vi "CRYTree Manipulate Sub.vi"(6 "Type":enum16{"Curves", "Values", "Results", "WFM"}(ring), 7 "sAction":string, 8 "sData":string[](array[string]), 9 "nData":i32[](array[numeric]), 10 "sOption":string, 11 "Tree in":refnum<vi>) -> (0 "bData out":bool, 1 "sData Out":string[](array[string]), 2 "bOnlyGroup":bool, 3 "Tree Out":refnum<vi>, 4 "bCategory":bool)   [LabVIEW 2013]
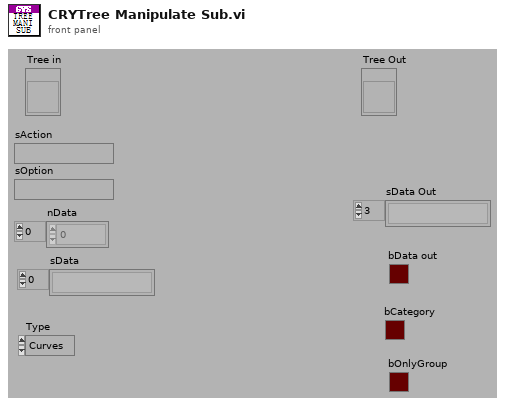
[diagram p1: front panel]
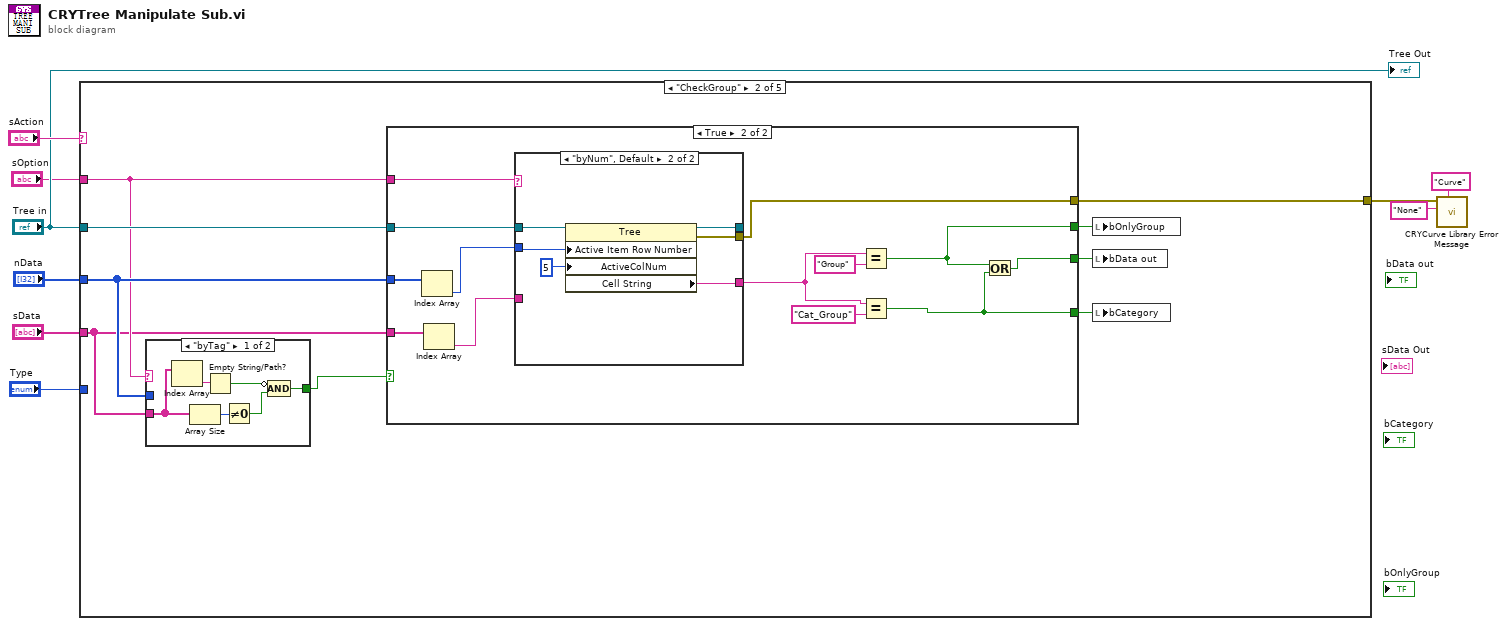
[diagram p0: block diagram]
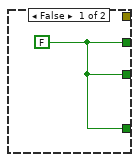
[diagram p3: hidden frame]
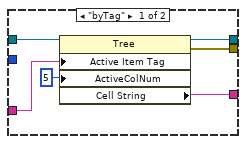
[diagram p4: hidden frame]
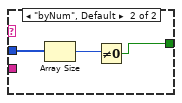
[diagram p5: hidden frame]
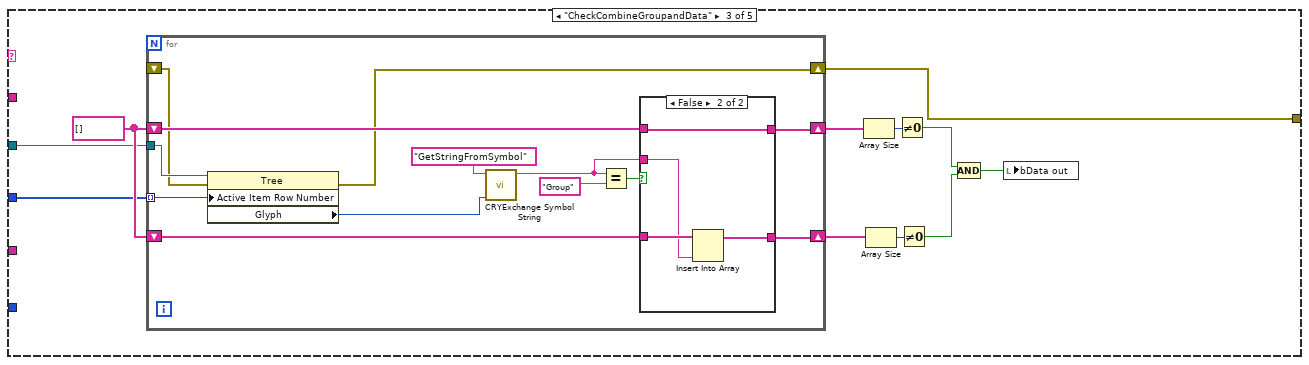
[diagram p6: hidden frame]
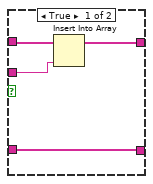
[diagram p7: hidden frame]
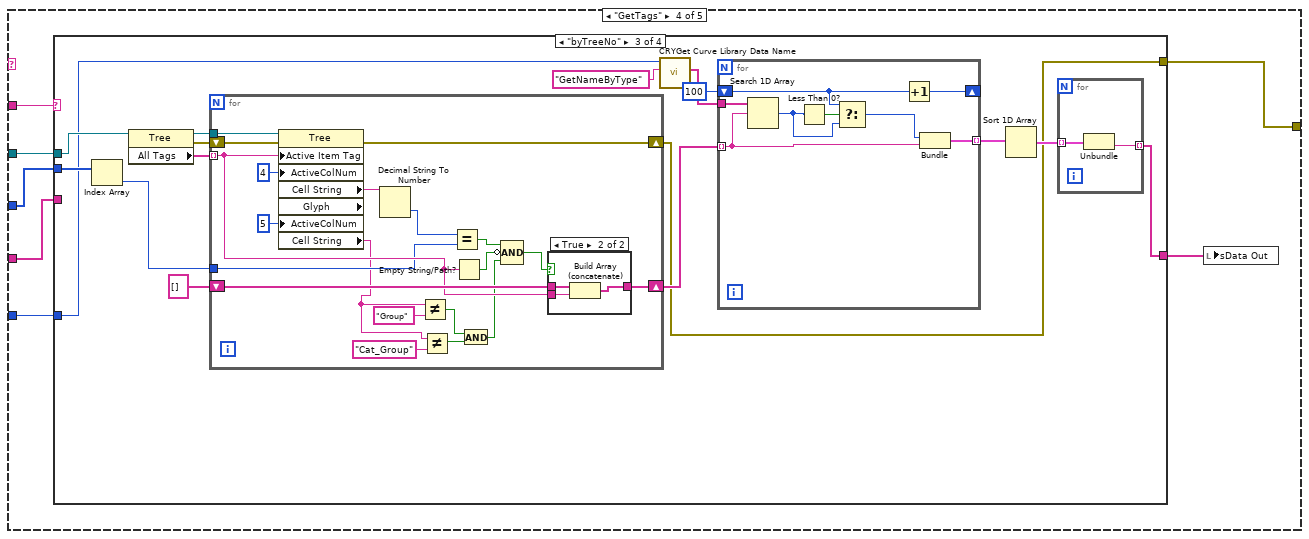
[diagram p8: hidden frame]
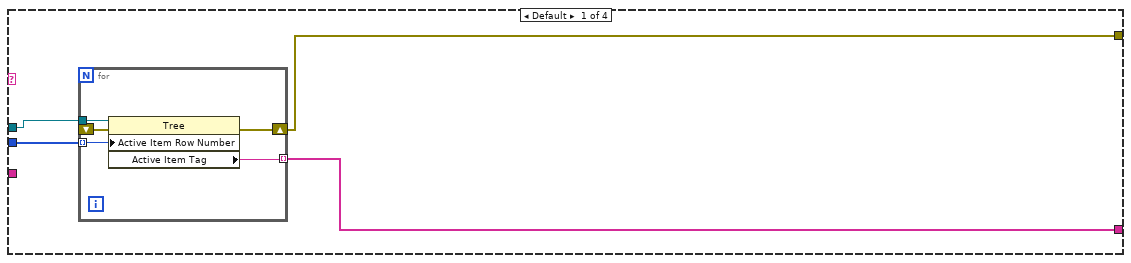
[diagram p9: hidden frame]
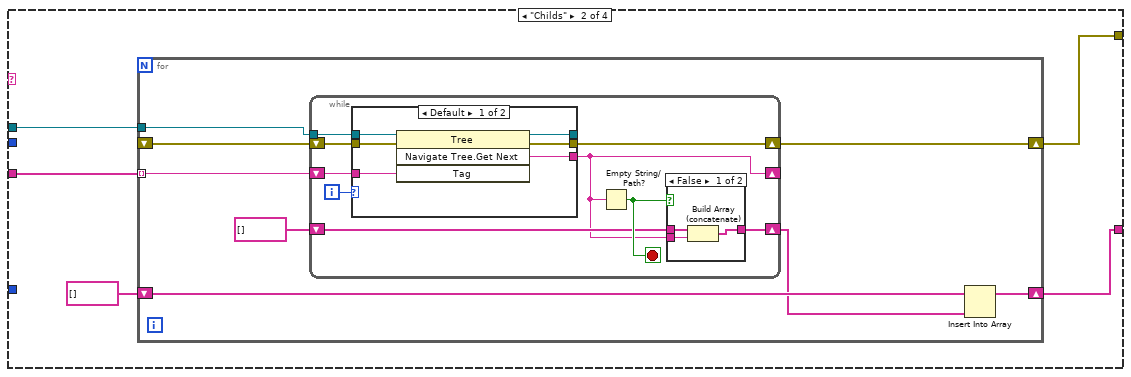
[diagram p10: hidden frame]
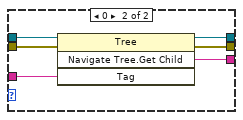
[diagram p12: hidden frame]
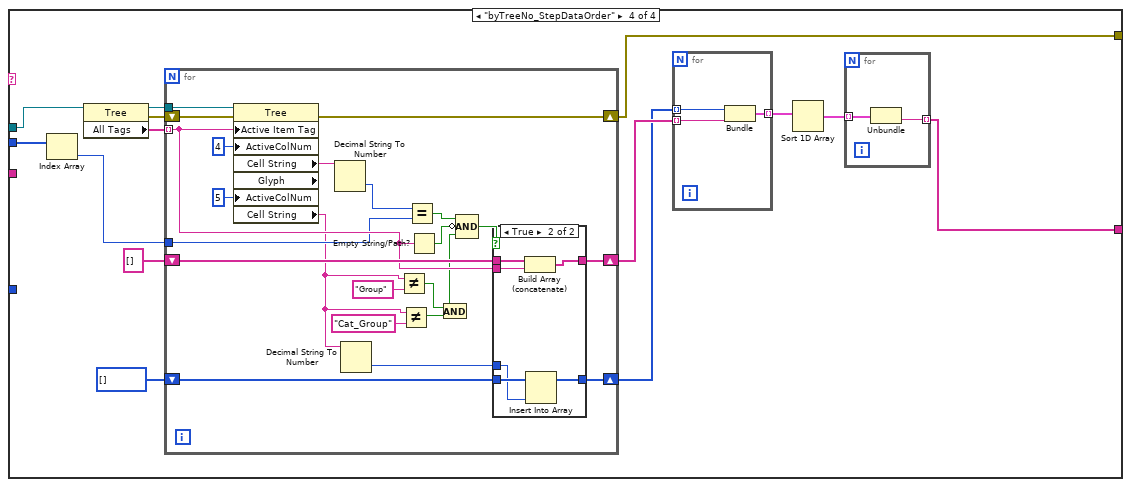
[diagram p14: hidden frame]
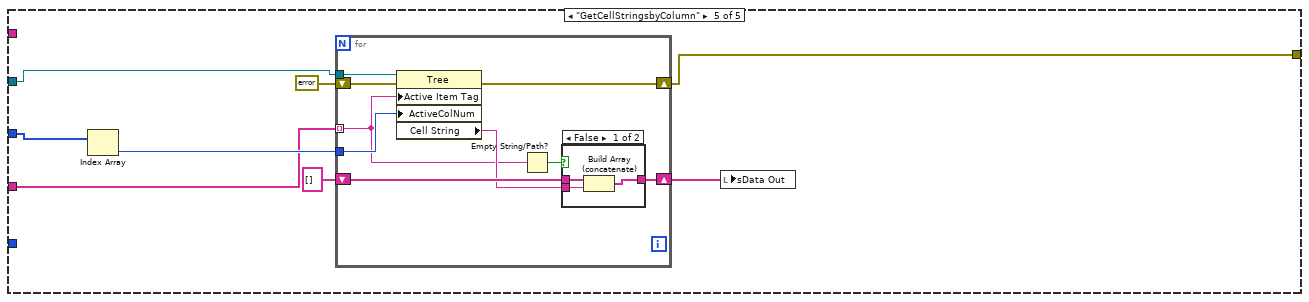
[diagram p16: hidden frame]
diagram:
  n1 = case shown="\"CheckGroup\"" "sAction" {
    tunnel: "nData" -> [_ w14 w55 w91 w245]
    tunnel: "Tree in" -> [_ w18 w56 w90 w242]
    tunnel: "sData" -> [_ w12 _ w89 w243]
    tunnel: "sOption" -> [_ w13 _ w88 _]
    tunnel: "Type" -> [_ _ _ w87 _]
    tunnel: [_ w10 w54 w86 w240] -> w1
    frame Default {
    }
    frame "CheckGroup" {
      n2 = case shown="\"byTag\"" w13 {
        tunnel: w12 -> [w48 _]
        tunnel: [w45 w51] -> w11
        tunnel: w14 -> [_ w53]
        frame "byTag" {
          n3 = Index Array(array=w48) -> (element=w49:string)  [unwired: 1 in]
          n4 = Array Size(array=w48) -> (size(s)=w47:i32)
          n5 = Empty String/Path?(string/path=w49) -> (empty?=w50:bool)
          n6 = Not Equal To 0?(x=w47) -> (x != 0?=w46:bool)
          n7 = Compound Arithmetic op=AND(invert w50, w46) -> (w45:bool)
        }
        frame "byNum", Default {
          n8 = Array Size(array=w53) -> (size(s)=w52:i32)
          n9 = Not Equal To 0?(x=w52) -> (x != 0?=w51:bool)
        }
      }
      n10 = case shown="True" w11 {
        tunnel: w18 -> [_ w31]
        tunnel: w13 -> [_ w30]
        tunnel: [w19 w29] -> w17
        tunnel: [w19 w27] -> w16
        tunnel: [w19 w26] -> w15
        tunnel: w12 -> [_ w22]
        tunnel: w14 -> [_ w21]
        tunnel: [_ w20] -> w10
        frame False {
          w19 = FALSE
        }
        frame True {
          n11 = Index Array(array=w21) -> (element=w25:i32)  [unwired: 1 in]
          n12 = Index Array(array=w22) -> (element=w24:string)  [unwired: 1 in]
          n13 = case shown="\"byNum\", Default" w30 {
            tunnel: w31 -> [w38 w44]
            tunnel: [w37 w43] -> _
            tunnel: w25 -> [_ w40]
            tunnel: [w35 w41] -> w23
            tunnel: w24 -> [w34 _]
            tunnel: [w33 w39] -> w20
            frame "byTag" {
              n14 = property class="Tree"(reference=w38, "Active Item Tag"=w34, "ActiveColNum"=5 ("Active Cell:Active Column Number")) -> (reference out=w37:refnum<vi>, error out=w33:errorcluster, "Cell String"=w35:string)  [unwired: 1 in]
            }
            frame "byNum", Default {
              n15 = property class="Tree"(reference=w44, "Active Item Row Number"=w40, "ActiveColNum"=5 ("Active Cell:Active Column Number")) -> (reference out=w43:refnum<vi>, error out=w39:errorcluster, "Cell String"=w41:string)  [unwired: 1 in]
            }
          }
          n16 = Equal?(x=w23, y="Group" ("sData out")) -> (x = y?=w29:bool)
          n17 = Equal?(x=w23, y="Cat_Group" ("sData out")) -> (x = y?=w26:bool)
          n18 = Or(x=w29, y=w26) -> (x .or. y?=w27:bool)
        }
      }
      n19 = local write "bOnlyGroup"(w17) -> ()
      n20 = local write "bData out"(w16) -> ()
      n21 = local write "bCategory"(w15) -> ()
    }
    frame "CheckCombineGroupandData" {
      w64 = string[] []
      n22 = for {
        tunnel: w55 -> [w71] mode=indexing
        shift-right: [w74] -> w63
        shift-left: w64 -> [w75]
        shift-right: [w72] -> w60
        shift-left: w64 -> [w73]
        tunnel: w56 -> [w69]
        shift-right: [w66] -> w54
        shift-left: _ -> [w65]
        n23 = property class="Tree"(reference=w69, error in=w65, "Active Item Row Number"=w71) -> (error out=w66:errorcluster, "Glyph"=w70:i32)  [unwired: 1 out]
        n24 = call "CRYExchange Symbol String.vi"("nData"=w70, "sAction"="GetStringFromSymbol") -> ("sData out"=w68:string)  [unwired: 8 in, 1 out]
        n25 = Equal?(x=w68, y="Group" ("sData out")) -> (x = y?=w67:bool)
        n26 = case shown="False" w67 {
          tunnel: w68 -> [w79 w83]
          tunnel: w75 -> [w81 w82]
          tunnel: [w80 w82] -> w74
          tunnel: w73 -> [w78 w85]
          tunnel: [w78 w84] -> w72
          frame True {
            n27 = Insert Into Array(array=w81, new element=w79) -> (w80:string[])  [unwired: 1 in]
          }
          frame False {
            n28 = Insert Into Array(array=w85, new element=w83) -> (w84:string[])  [unwired: 1 in]
          }
        }
      }
      n29 = Array Size(array=w63) -> (size(s)=w62:i32)
      n30 = Array Size(array=w60) -> (size(s)=w61:i32)
      n31 = Not Equal To 0?(x=w62) -> (x != 0?=w59:bool)
      n32 = Not Equal To 0?(x=w61) -> (x != 0?=w58:bool)
      n33 = Compound Arithmetic op=AND(w59, w58) -> (w57:bool)
      n34 = local write "bData out"(w57) -> ()
    }
    frame "GetTags" {
      n35 = case shown="\"byTreeNo\"" w88 {
        tunnel: [w95 w106 w144 w194] -> w92
        tunnel: w91 -> [w94 _ w155 w203]
        tunnel: w90 -> [w96 w105 w152 w200]
        tunnel: w89 -> [_ w104 _ _]
        tunnel: w87 -> [_ _ w143 _]
        tunnel: [w93 w102 w141 w190] -> w86
        frame Default {
          n36 = for {
            tunnel: w96 -> [w101]
            tunnel: w94 -> [w100] mode=indexing
            tunnel: [w99] -> w95 mode=indexing
            shift-right: [w98] -> w93
            shift-left: _ -> [w97]
            n37 = property on="Property Node" class="Tree"(reference=w101, error in=w97, "Active Item Row Number"=w100) -> (error out=w98:errorcluster, "Active Item Tag"=w99:string)  [unwired: 1 out]
          }
        }
        frame "Childs" {
          n38 = for {
            tunnel: w105 -> [w113]
            tunnel: w104 -> [w112] mode=indexing
            shift-right: [w109] -> w106
            shift-left: string[] [] -> [w111]
            shift-right: [w108] -> w102
            shift-left: _ -> [w107]
            n39 = while {
              tunnel: w113 -> [w123]
              shift-right: [w115] -> _
              shift-left: w112 -> [w122]
              shift-right: [w118] -> w108
              shift-left: w107 -> [w121]
              shift-right: [w117] -> w110
              shift-left: string[] [] -> [w116]
              i -> [w120]
              stop <- w119 stop-if-true
              n40 = case shown="Default" w120 {
                tunnel: w123 -> [w133 w139]
                tunnel: w122 -> [w132 w138]
                tunnel: [w130 w137] -> w115
                tunnel: w121 -> [w131 w136]
                tunnel: [w129 w135] -> w118
                tunnel: [w128 w134] -> _
                frame Default {
                  n41 = invoke class="Tree" method="Navigate Tree.Get Next"(reference=w133, error in=w131, "Tag"=w132) -> (reference out=w128:refnum<vi>, error out=w129:errorcluster, "Navigate Tree:Get Next Item"=w130:string)  [unwired: 1 in, 1 out]
                }
                frame 0 {
                  n42 = invoke class="Tree" method="Navigate Tree.Get Child"(reference=w139, error in=w136, "Tag"=w138) -> (reference out=w134:refnum<vi>, error out=w135:errorcluster, "Navigate Tree:Get Child"=w137:string)  [unwired: 1 in, 1 out]
                }
              }
              n43 = Empty String/Path?(string/path=w115) -> (empty?=w119:bool)
              n44 = case shown="False" w119 {
                tunnel: [w124 w127] -> w117
                tunnel: w116 -> [w126 w127]
                tunnel: w115 -> [w125 _]
                frame False {
                  n45 = Build Array (concatenate)(w126, w125) -> (w124:string[])
                }
                frame True {
                }
              }
            }
            n46 = Insert Into Array(array=w111, new element=w110) -> (w109:string[])  [unwired: 1 in]
          }
        }
        frame "byTreeNo" {
          n47 = Index Array(array=w155) -> (element=w150:i32)  [unwired: 1 in]
          n48 = property class="Tree"(reference=w152) -> (reference out=w151:refnum<vi>, error out=w140:errorcluster, "All Tags"=w153:string[])  [unwired: 1 in]
          n49 = for {
            tunnel: w151 -> [w182]
            shift-right: [w183] -> w141
            shift-left: w140 -> [w181]
            shift-right: [w184] -> w147
            shift-left: string[] [] -> [w185]
            tunnel: w153 -> [w180] mode=indexing
            tunnel: w150 -> [w179]
            n50 = property class="Tree" props=["Active Item Tag", "ActiveColNum", "Cell String", "Glyph", "ActiveColNum", "Cell String"](reference=w182, error in=w181, "Active Item Tag"=w180, "ActiveColNum"=4 ("Active Cell:Active Column Number"), "ActiveColNum"=5 ("Active Cell:Active Column Number")) -> (error out=w183:errorcluster, "Cell String"=w174:string, "Cell String"=w166:string)  [unwired: 2 out]
            n51 = Decimal String To Number(string=w174) -> (number=w173:i32)  [unwired: 2 in, 1 out]
            n52 = Not Equal?(x=w166, y="Group" ("sData out")) -> (x != y?=w170:bool)
            n53 = Not Equal?(x=w166, y="Cat_Group" ("sData out")) -> (x != y?=w169:bool)
            n54 = Equal?(x=w173, y=w179) -> (x = y?=w177:bool)
            n55 = Empty String/Path?(string/path=w180) -> (empty?=w178:bool)
            n56 = And(x=w170, y=w169) -> (x .and. y?=w168:bool)
            n57 = Compound Arithmetic op=AND(w177, invert w178, w168) -> (w176:bool)
            n58 = case shown="True" w176 {
              tunnel: w185 -> [w186 w189]
              tunnel: w180 -> [_ w188]
              tunnel: [w186 w187] -> w184
              frame False {
              }
              frame True {
                n59 = Build Array (concatenate)(w189, w188) -> (w187:string[])
              }
            }
          }
          n60 = call "CRYGet Curve Library Data Name.vi"("sAction"="GetNameByType", "Type"=w143) -> ("sNames"=w148:string[])  [unwired: 6 in, 3 out]
          n61 = for {
            tunnel: w148 -> [w165]
            tunnel: w147 -> [w164] mode=indexing
            tunnel: [w163] -> w146 mode=indexing
            shift-right: [w160] -> _
            shift-left: 100 ("index of element") -> [w161]
            n62 = Search 1D Array(1D array=w165, element=w164) -> (index of element=w159:i32)  [unwired: 1 in]
            n63 = Less Than 0?(x=w159) -> (x < 0?=w162:bool)
            n64 = Select(t=w161, s=w162, f=w159) -> (s? t:f=w158:i32)
            n65 = Increment(x=w161) -> (x+1=w160:i32)
            n66 = Bundle("index of element"=w158, w164) -> (w163:cluster{"index of element":i32, string})  [unwired: 1 in]
          }
          n67 = Sort 1D Array(array=w146) -> (sorted array=w145:cluster{"index of element":i32, string}[])
          n68 = for {
            tunnel: w145 -> [w157] mode=indexing
            tunnel: [w156] -> w144 mode=indexing
            n69 = Unbundle(w157) -> (w156:string)  [unwired: 1 out]
          }
        }
        frame "byTreeNo_StepDataOrder" {
          n70 = Index Array(array=w203) -> (element=w198:i32)  [unwired: 1 in]
          n71 = property class="Tree"(reference=w200) -> (reference out=w199:refnum<vi>, error out=w191:errorcluster, "All Tags"=w201:string[])  [unwired: 1 in]
          n72 = for {
            tunnel: w199 -> [w228]
            shift-right: [w229] -> w190
            shift-left: w191 -> [w227]
            shift-right: [w230] -> w197
            shift-left: string[] [] -> [w231]
            tunnel: w201 -> [w226] mode=indexing
            tunnel: w198 -> [w225]
            shift-right: [w209] -> w192
            shift-left: i32[] [] ("appended array") -> [w210]
            n73 = property class="Tree" props=["Active Item Tag", "ActiveColNum", "Cell String", "Glyph", "ActiveColNum", "Cell String"](reference=w228, error in=w227, "Active Item Tag"=w226, "ActiveColNum"=4 ("Active Cell:Active Column Number"), "ActiveColNum"=5 ("Active Cell:Active Column Number")) -> (error out=w229:errorcluster, "Cell String"=w220:string, "Cell String"=w212:string)  [unwired: 2 out]
            n74 = Decimal String To Number(string=w220) -> (number=w219:i32)  [unwired: 2 in, 1 out]
            n75 = Decimal String To Number(string=w212) -> (number=w211:i32)  [unwired: 2 in, 1 out]
            n76 = Not Equal?(x=w212, y="Group" ("sData out")) -> (x != y?=w216:bool)
            n77 = Not Equal?(x=w212, y="Cat_Group" ("sData out")) -> (x != y?=w215:bool)
            n78 = Equal?(x=w219, y=w225) -> (x = y?=w223:bool)
            n79 = Empty String/Path?(string/path=w226) -> (empty?=w224:bool)
            n80 = And(x=w216, y=w215) -> (x .and. y?=w214:bool)
            n81 = Compound Arithmetic op=AND(w223, invert w224, w214) -> (w222:bool)
            n82 = case shown="True" w222 {
              tunnel: w231 -> [w233 w239]
              tunnel: w226 -> [_ w238]
              tunnel: [w233 w237] -> w230
              tunnel: w211 -> [_ w234]
              tunnel: w210 -> [w232 w236]
              tunnel: [w232 w235] -> w209
              frame False {
              }
              frame True {
                n83 = Build Array (concatenate)(w239, w238) -> (w237:string[])
                n84 = Insert Into Array(array=w236, new element=w234) -> (w235:i32[])  [unwired: 1 in]
              }
            }
          }
          n85 = for {
            tunnel: w197 -> [w206] mode=indexing
            tunnel: [w208] -> w196 mode=indexing
            tunnel: w192 -> [w207] mode=indexing
            n86 = Bundle(w207, w206) -> (w208:cluster{i32, string})  [unwired: 1 in]
          }
          n87 = Sort 1D Array(array=w196) -> (sorted array=w195:cluster{i32, string}[])
          n88 = for {
            tunnel: w195 -> [w205] mode=indexing
            tunnel: [w204] -> w194 mode=indexing
            n89 = Unbundle(w205) -> (w204:string)  [unwired: 1 out]
          }
        }
      }
      n90 = local write "sData Out"(w92) -> ()
    }
    frame "GetCellStringsbyColumn" {
      n91 = Index Array(array=w245) -> (element=w244:i32)  [unwired: 1 in]
      n92 = for {
        tunnel: w242 -> [w250]
        shift-right: [w253] -> w240
        shift-left: errorcluster {"status"=FALSE, "code"=0, "source"=""} ("Fehler (Ausgang)") -> [w249]
        shift-right: [w254] -> w241
        shift-left: string[] [] -> [w255]
        tunnel: w244 -> [w251]
        tunnel: w243 -> [w248] mode=indexing
        n93 = property class="Tree"(reference=w250, error in=w249, "Active Item Tag"=w248, "ActiveColNum"=w251) -> (error out=w253:errorcluster, "Cell String"=w252:string)  [unwired: 1 out]
        n94 = Empty String/Path?(string/path=w248) -> (empty?=w256:bool)
        n95 = case shown="False" w256 {
          tunnel: w255 -> [w259 w260]
          tunnel: w252 -> [w258 _]
          tunnel: [w257 w260] -> w254
          frame False {
            n96 = Build Array (concatenate)(w259, w258) -> (w257:string[])
          }
          frame True {
          }
        }
      }
      n97 = local write "sData Out"(w241) -> ()
    }
  }
  n98 = call "CRYCurve Library Error Message.vi"("sAction"="Curve", "sOption"="None", "error IO"=w1) -> ()  [unwired: 9 in]
  "Tree Out" <- "Tree in"
